vi "old tests.vi"() -> ()   [LabVIEW 2018]
uses:
  CCDCamera/CCDCamera.lvclass
  <userlib>/atmcd32d.llb/Shutter_mode typedef.ctl
  <userlib>/atmcd32d.llb/ReadMode_mode typedef.ctl
  <userlib>/atmcd32d.llb/AcquisitionMode_mode typedef.ctl
  TCPIP/TCPIP.lvclass
  <userlib>/atmcd32d.llb/FITS_type typedef.ctl
  Simulated_CCD_Camera/Simulated_CCD_Camera.lvclass
  Interface/Interface.lvclass
  <userlib>/gfitsio/gfitsio.lvlib
  <userlib>/gfitsio/cfitsio-bitpix.ctl
  C:/Users/observer/Desktop/SPARC4_ACS/SPARC4_ACS/Simulated_CCD_Camera/Simulated_CCD_Camera.lvclass
  <vilib>/Enthought/Python Integration Toolkit/Python Integration Toolkit.lvlib
  <vilib>/Enthought/Python Integration Toolkit/api/Unpack String.vi
  <userlib>/gfitsio/gfitsio-write-image-subset-variant.vi
panel:
  out "error out 7":errorcluster
  in  "Previous CCD Config 2":T4={"PREAMP"=enum."Gain 1", "READOUT_RATE"=enum."1 MHz", "EM_GAIN"=2, "VBIN"=1, "INITIAL_LINE"=1, "INITIAL_COLUMN"=1, "FINAL_LINE"=1024, "FINAL_COLUMN"=1024, "TRIGGER_MODE"=enum."Internal", "HBIN"=1, "SHUTTER_TTL"=enum."TTL Low", "SHUTTER_MODE"=enum."Close", "SHUTTER_OPENING_TIME"=50, "SHUTTER_CLOSING_TIME"=50, "VERTICAL_SHIFT_SPEED"=3, "READ_MODE"=enum."Image", "FRAME_TRANSFER"=TRUE, "VERTICAL_CLOCK_VOLTAGE"=enum."0", "ACQUISITION_MODE"=enum."Kinetics", "AD_CHANNEL"=0, "EM_MODE"=enum."Electron Multiplying"}
  in  "Previous SET parameters 2":T5={"COOLER_POWER_STATUS"=0, "TEMP"=20, "EXPTIME"=1.0, "#FRAMES"=1, "#CUBES"=1}
  out "error out 6":errorcluster
  out "Array":string[](array[string])
  out "Value":string
  out "error out 5":errorcluster
  out "data out":string
  out "Message":string
  out "error out 4":errorcluster
  out "error out 3":errorcluster
  in  "TCPIP in":refnum<class "TCPIP.lvclass">
  out "error out 2":errorcluster
  out "error out":errorcluster
  in  "Previous SET parameters":T5
  in  "Previous CCD Config":T4={"PREAMP"=enum."Gain 1", "READOUT_RATE"=enum."1 MHz", "EM_GAIN"=2, "VBIN"=1, "INITIAL_LINE"=1, "INITIAL_COLUMN"=1, "FINAL_LINE"=1024, "FINAL_COLUMN"=1024, "TRIGGER_MODE"=enum."Internal", "HBIN"=1, "SHUTTER_TTL"=enum."TTL Low", "SHUTTER_MODE"=enum."Close", "SHUTTER_OPENING_TIME"=50, "SHUTTER_CLOSING_TIME"=50, "VERTICAL_SHIFT_SPEED"=3, "READ_MODE"=enum."Image", "FRAME_TRANSFER"=TRUE, "VERTICAL_CLOCK_VOLTAGE"=enum."0", "ACQUISITION_MODE"=enum."Kinetics", "AD_CHANNEL"=0, "EM_MODE"=enum."Electron Multiplying"}
  in  "CCDCamera.lvclass":refnum<class "CCDCamera.lvclass">
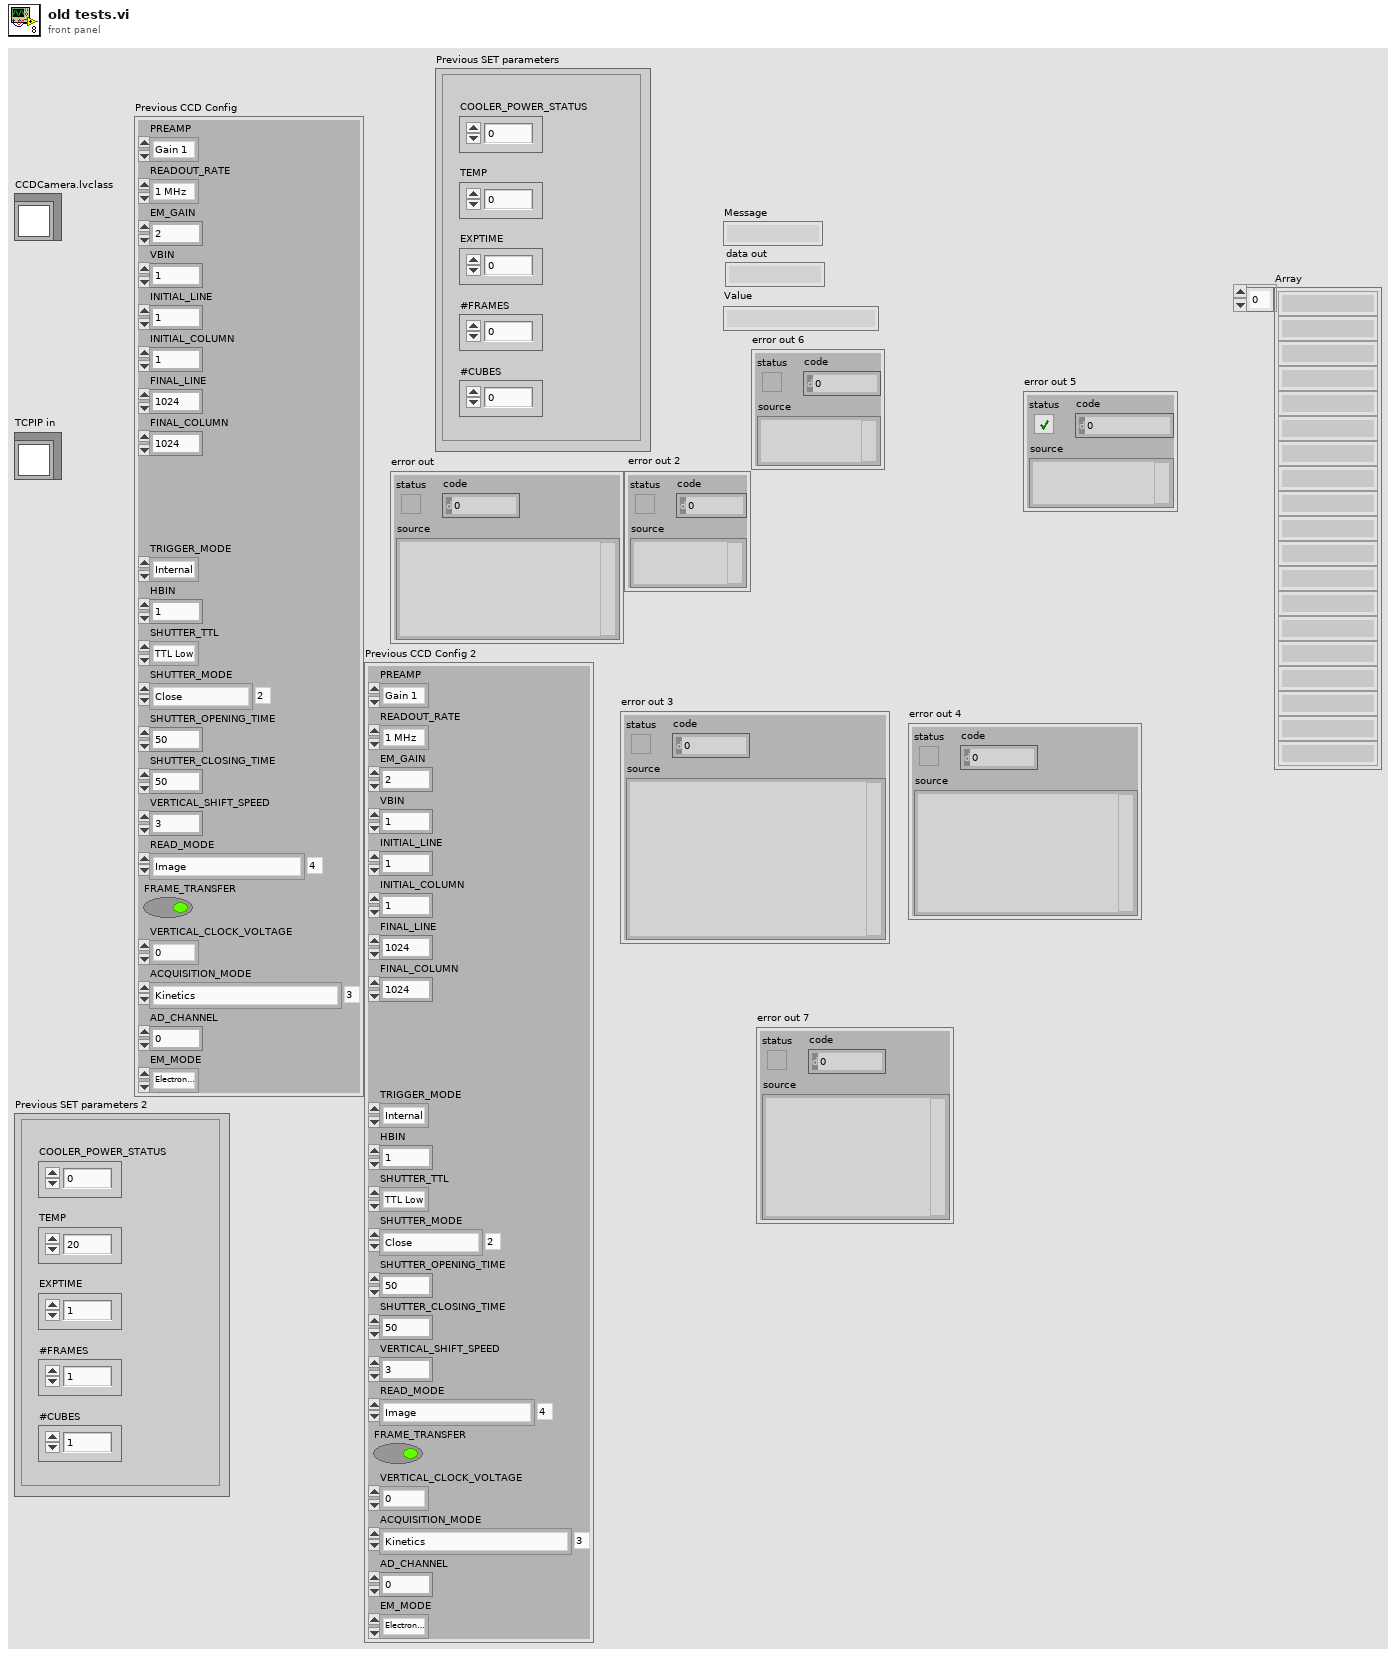
[diagram p1: front panel]
types:
  T1 = typedef "Shutter_mode typedef.ctl" = enum16{"Auto", "Open", "Close", "N/A (3)", "Open FVB Series", "Open Any Series"}
  T2 = typedef "ReadMode_mode typedef.ctl" = enum16{"Full Vertical Binning", "Multi-Track", "Random-Track", "Single-Track", "Image"}
  T3 = typedef "AcquisitionMode_mode typedef.ctl" = enum16{"Reserved (0)", "Single Scan", "Accumulate", "Kinetics", "Fast Kinetics", "Run Till Abort", "Reserved (6)", "Reserved (7)", "Reserved (8)", "Time Delayed Integration"}
  T4 = cluster{"PREAMP":enum16{"Gain 1", "Gain 2"}, "READOUT_RATE":enum16{"30 MHz", "20 MHz", "10 MHz", "1 MHz"}, "EM_GAIN":u16, "VBIN":u16, "INITIAL_LINE":u16, "INITIAL_COLUMN":u16, "FINAL_LINE":u16, "FINAL_COLUMN":u16, "TRIGGER_MODE":enum16{"Internal", "External", "N/A", "N/A_1", "N/A_2", "N/A_3", "External Start"}, "HBIN":u16, "SHUTTER_TTL":enum16{"TTL Low", "TTL High"}, "SHUTTER_MODE":T1, "SHUTTER_OPENING_TIME":u16, "SHUTTER_CLOSING_TIME":u16, "VERTICAL_SHIFT_SPEED":u16, "READ_MODE":T2, "FRAME_TRANSFER":bool, "VERTICAL_CLOCK_VOLTAGE":enum16{"0", "+1", "+2", "+3", "+4"}, "ACQUISITION_MODE":T3, "AD_CHANNEL":u16, "EM_MODE":enum16{"Electron Multiplying", "Conventional"}}
  T5 = cluster{"COOLER_POWER_STATUS":u16, "TEMP":i32, "EXPTIME":dbl, "#FRAMES":u32, "#CUBES":u32}
  T6 = typedef "FITS_type typedef.ctl" = enum16{"Unsigned 16", "Unsigned 32", "Signed 16", "Signed 32", "Float"}
  T7 = enum16{"open", "open or create", "create or replace", "create", "open (read only)"}
  T8 = typedef "gfitsio.lvlib/cfitsio-bitpix.ctl" = i32
  T9 = typedef "gfitsio.lvlib/gfitsio-refnum.ctl" = refnum<k1>
  T10 = enum16{"Standard", "Buffered", "CRLF", "Immediate"}
  T11 = typedef "Python Integration Toolkit.lvlib/Session ID.ctl" = u64
  T12 = typedef "Python Integration Toolkit.lvlib/Python Objects.ctl" = variant
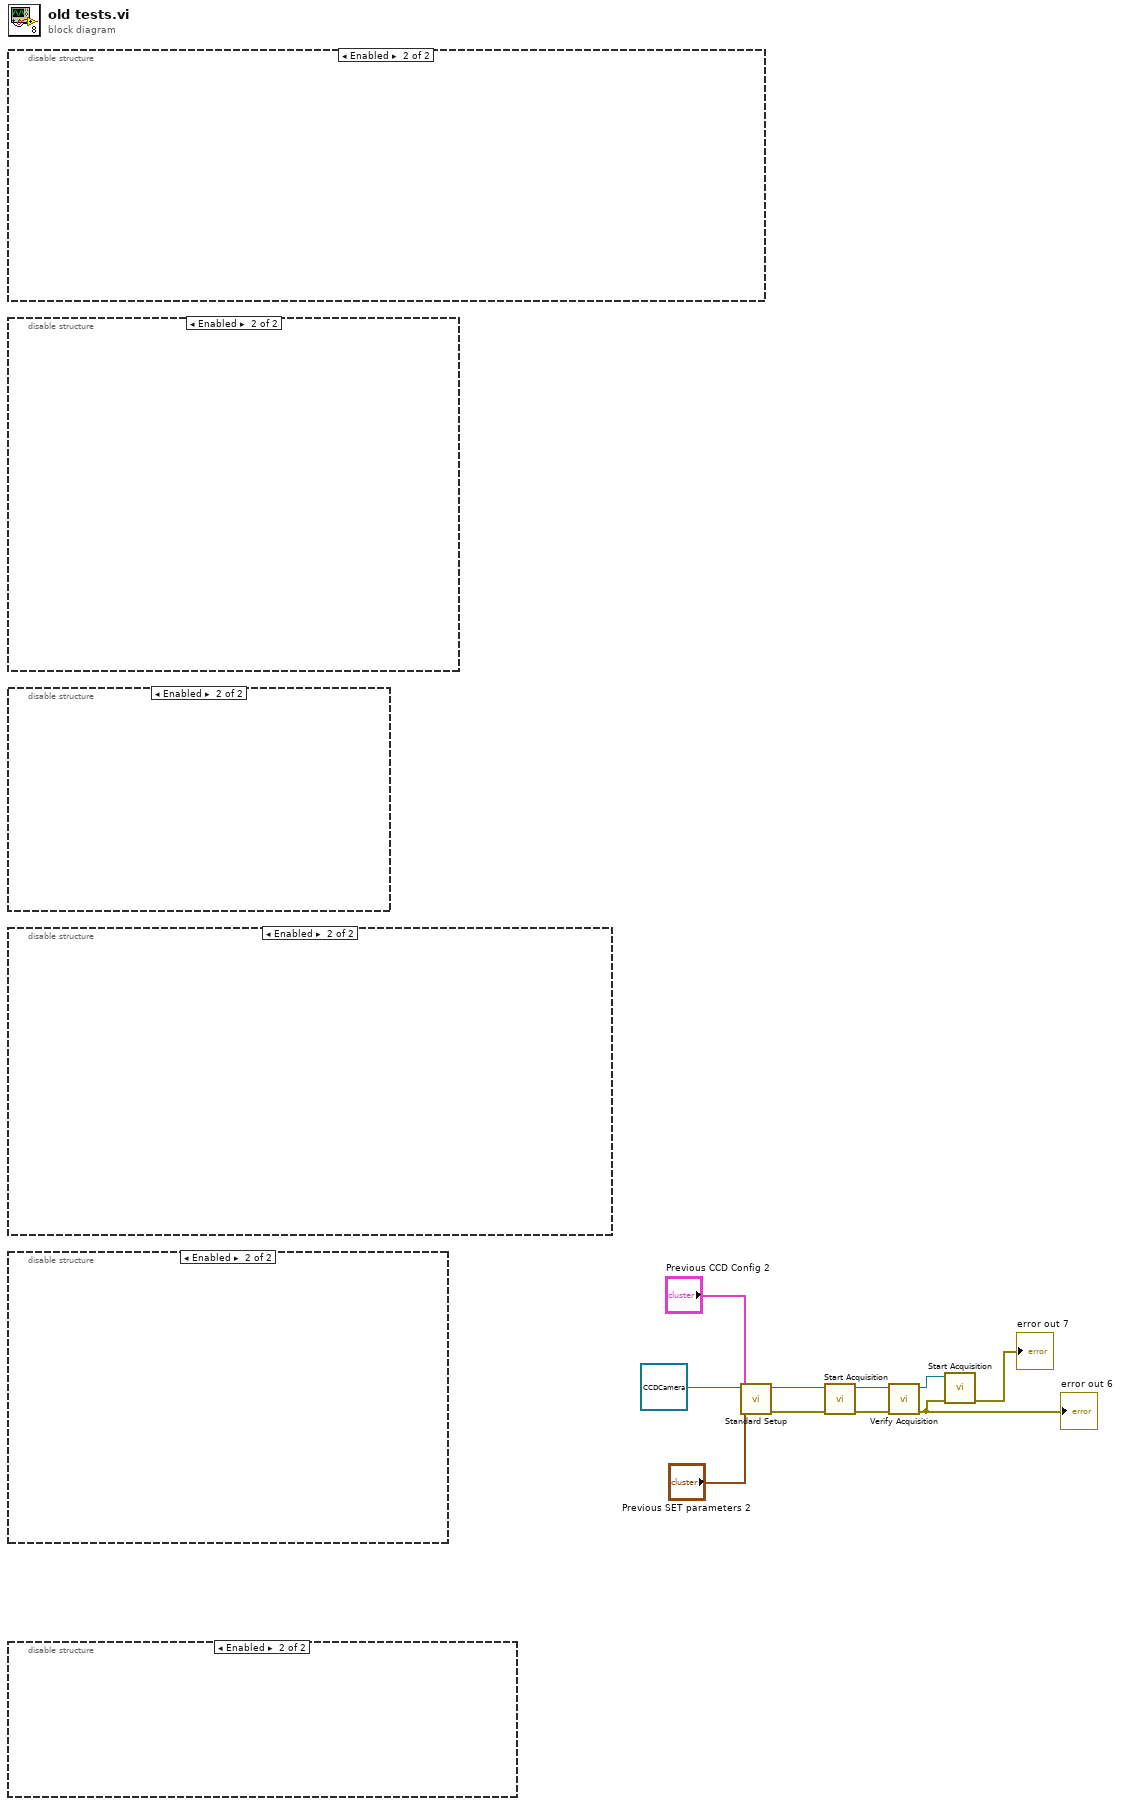
[diagram p0: block diagram]
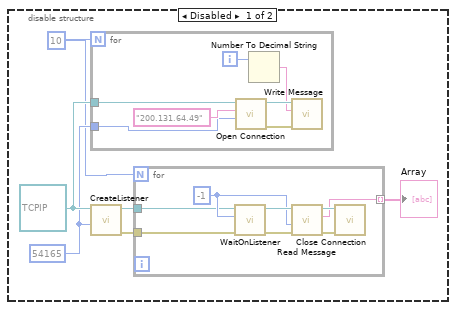
[diagram p2: hidden frame]
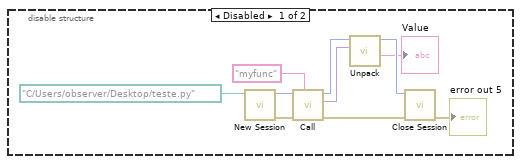
[diagram p3: hidden frame]
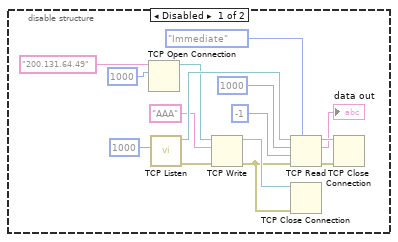
[diagram p4: hidden frame]
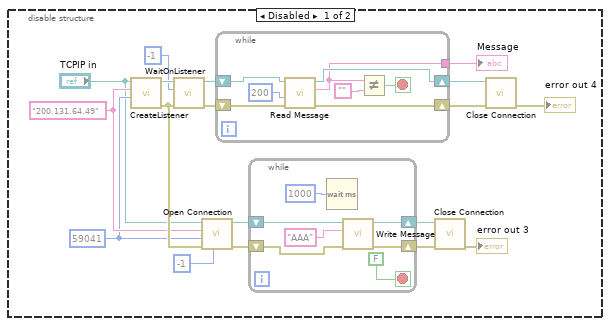
[diagram p5: hidden frame]
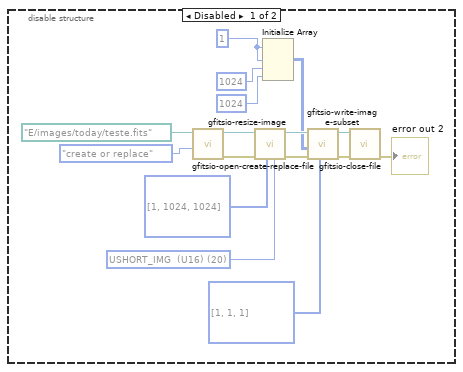
[diagram p6: hidden frame]
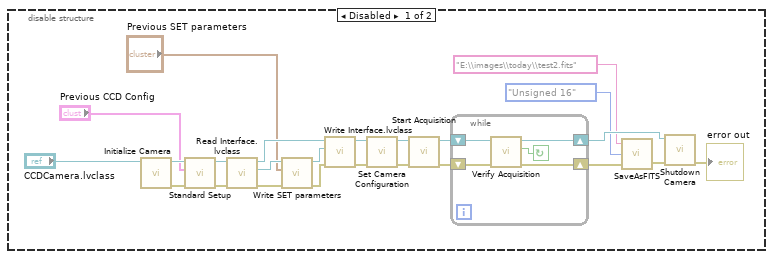
[diagram p7: hidden frame]
diagram:
  n1 = disable-structure shown="Enabled" {
    frame Disabled {
      n2 = call-dynamic "Initialize Camera.vi"("CCDCamera in"="CCDCamera.lvclass") -> ("error out"=w30:errorcluster, "CCDCamera out"=w34:refnum<class "CCDCamera.lvclass">)  [unwired: 9 in]
      n3 = call-dynamic "Standard Setup.vi"("error in (no error)"=w30, "Previous CCD Config"="Previous CCD Config", "CCDCamera in"=w34) -> ("error out"=w21:errorcluster, "CCDCamera out"=w25:refnum<class "CCDCamera.lvclass">)  [unwired: 7 in]
      n4 = call "Read Interface.lvclass.vi"("error in (no error)"=w21, "Simulated_CCD_Camera in"=w25) -> ("error out"=w20:errorcluster, "Interface.lvclass"=w17:refnum<class "Interface.lvclass">, "Simulated_CCD_Camera out"=w24:refnum<class "CCDCamera.lvclass">)  [unwired: 7 in]
      n5 = call "Write SET parameters.vi"("error in (no error)"=w20, "SET parameters"="Previous SET parameters", "Interface in"=w17) -> ("error out"=w19:errorcluster, "Interface out"=w18:refnum<class "Interface.lvclass">)  [unwired: 7 in]
      n6 = call "Write Interface.lvclass.vi"("error in (no error)"=w19, "Interface.lvclass"=w18, "Simulated_CCD_Camera in"=w24) -> ("error out"=w22:errorcluster, "Simulated_CCD_Camera out"=w23:refnum<class "CCDCamera.lvclass">)  [unwired: 7 in]
      n7 = call-dynamic "Set Camera Configuration.vi"("error in (no error)"=w22, "CCDCamera in"=w23) -> ("error out"=w26:errorcluster, "CCDCamera out"=w27:refnum<class "CCDCamera.lvclass">)  [unwired: 8 in]
      n8 = call-dynamic "Start Acquisition.vi"("error in (no error)"=w26, "CCDCamera in"=w27) -> ("error out"=w31:errorcluster, "CCDCamera out"=w33:refnum<class "CCDCamera.lvclass">)  [unwired: 8 in]
      n9 = while {
        shift-right: [w38] -> w32
        shift-left: w33 -> [w39]
        shift-right: [w35] -> w11
        shift-left: w31 -> [w37]
        stop <- w36 continue-if-true
        n10 = call-dynamic "Verify Acquisition.vi"("error in (no error)"=w37, "CCDCamera in"=w39) -> ("error out"=w35:errorcluster, "Acquiring"=w36:bool, "CCDCamera out"=w38:refnum<class "CCDCamera.lvclass">)  [unwired: 7 in]
      }
      n11 = call <userlib>:"SaveAsFITS.vi"("error in (no error)"=w11, "FITS_type"=FITS_type_typedef."Unsigned 16", "path"="E:\\images\\today\\test2.fits") -> ("error out"=w12:errorcluster)  [unwired: 1 out]
      n12 = call-dynamic "Shutdown Camera.vi"("error in (no error)"=w12, "CCDCamera in"=w32) -> ("error out"=→"error out":errorcluster)  [unwired: 8 in, 1 out]
    }
    frame Enabled {
    }
  }
  n13 = disable-structure shown="Enabled" {
    frame Disabled {
      w45 = 1 ("dimension size")
      w48 = T8 20 items=["<invalid type>"=0, "BYTE_IMG  (U8)"=8, "SHORT_IMG  (I16)"=16, "USHORT_IMG  (U16)"=20, "LONG_IMG  (I32)"=32, "ULONG_IMG  (U32)"=40, "FLOAT_IMG  (SGL)"=-32, "DOUBLE_IMG  (DBL)"=-64] ("image data type")
      n14 = call <userlib>:"gfitsio-open-create-replace-file.vi"("function (open)"=T7."create or replace", "file path (dialog if empty)"=path "E:/images/today/teste.fits") -> ("error out"=w50:errorcluster, "gfits refnum"=w55:T9)  [unwired: 7 in, 1 out]
      n15 = call <userlib>:"gfitsio-resize-image.vi"("image data type"=w48, "naxes"=i32[] [1, 1024, 1024], "error in (no error)"=w50, "gfits refnum"=w55) -> ("error out"=w51:errorcluster, "dup gfits refnum"=w54:T9)  [unwired: 6 in]
      n16 = Initialize Array(w45, w45, 1024 ("dimension size"), 1024 ("dimension size")) -> (w44:i32[][][])
      n17 = call-poly <userlib>:"gfitsio-write-image-subset.vi"("fpixel"=i32[] [1, 1, 1] ("naxes"), "error in (no error)"=w51, "data"=w44, "gfits refnum"=w54) -> ("error out"=w52:errorcluster, "dup gfits refnum"=w53:T9)  [unwired: 6 in]
      n18 = call <userlib>:"gfitsio-close-file.vi"("error in (no error)"=w52, "gfits refnum"=w53) -> ("error out"=→"error out 2":errorcluster)  [unwired: 8 in, 1 out]
    }
    frame Enabled {
    }
  }
  n19 = disable-structure shown="Enabled" {
    frame Disabled {
      n20 = TCP Open Connection(address="200.131.64.49", remote port or service name=u16 1000) -> (connection ID=w64:refnum<k5>)  [unwired: 3 in, 1 out]
      n21 = call <vilib>:"TCP Listen.vi"("port"=u16 1000) -> ("error out"=w59:errorcluster, "connection ID"=w69:refnum<k5>)  [unwired: 6 in, 3 out]
      n22 = TCP Write(connection ID=w64, data in="AAA", error in (no error)=w59) -> (connection ID out=w63:refnum<k5>, error out=w58:errorcluster)  [unwired: 1 in, 1 out]
      n23 = TCP Read(connection ID=w69, bytes to read=1000, error in (no error)=w58, 7:T10."Immediate" ("mode (standard)"), 9:-1 ("timeout ms (25000)")) -> (connection ID out=w68:refnum<k5>, data out=→"data out":string, error out=w67:errorcluster)
      n24 = TCP Close Connection(connection ID=w63, error in (no error)=w58) -> ()  [unwired: 1 in, 2 out]
      n25 = TCP Close Connection(connection ID=w68, error in (no error)=w67) -> ()  [unwired: 1 in, 2 out]
    }
    frame Enabled {
    }
  }
  n26 = disable-structure shown="Enabled" {
    frame Disabled {
      w85 = u16 59041 ("remote port")
      w86 = "200.131.64.49" ("IP")
      n27 = call-dynamic "CreateListener.vi"("remote port"=w85, 10:w86, "TCPIP in"="TCPIP in") -> ("error out"=w87:errorcluster, "TCPIP out"=w88:refnum<class "TCPIP.lvclass">)  [unwired: 7 in]
      n28 = call-dynamic "WaitOnListener.vi"("error in (no error)"=w87, "timeout ms"=-1, "TCPIP in"=w88) -> ("error out"=w76:errorcluster, "TCPIP out"=w77:refnum<class "TCPIP.lvclass">)  [unwired: 7 in]
      n29 = call "Open Connection.vi"("timeout"=-1, "error in (no error)"=w87, "remote port"=w85, "IP"=w86, "TCPIP in"="TCPIP in") -> ("error out"=w78:errorcluster, "TCPIP out"=w81:refnum<class "TCPIP.lvclass">)  [unwired: 5 in]
      n30 = while {
        tunnel: [w90] -> w72
        shift-right: [w92] -> w74
        shift-left: w77 -> [w96]
        shift-right: [w93] -> w75
        shift-left: w76 -> [w95]
        stop <- w91 stop-if-true
        n31 = call "Read Message.vi"("error in (no error)"=w95, "timeout"=200, "TCPIP in"=w96) -> ("error out"=w93:errorcluster, "Message"=w90:string, "TCPIP out"=w92:refnum<class "TCPIP.lvclass">)  [unwired: 6 in]
        n32 = Not Equal?(x=w90, y="") -> (x != y?=w91:bool)
      }
      "Message" <- w72
      n33 = while {
        shift-right: [w102] -> w80
        shift-left: w81 -> [w103]
        shift-right: [w101] -> w79
        shift-left: w78 -> [w100]
        stop <- FALSE stop-if-true
        n34 = Wait (ms)(milliseconds to wait=u32 1000) -> ()  [unwired: 1 out]
        n35 = call "Write Message.vi"("error in (no error)"=w100, "Message"="AAA", "TCPIP in"=w103) -> ("error out"=w101:errorcluster, "TCPIP out"=w102:refnum<class "TCPIP.lvclass">)  [unwired: 7 in]
      }
      n36 = call "Close Connection.vi"("error in (no error)"=w79, "TCPIP in"=w80) -> ("error out"=→"error out 3":errorcluster)  [unwired: 8 in, 1 out]
      n37 = call "Close Connection.vi"("error in (no error)"=w75, "TCPIP in"=w74) -> ("error out"=→"error out 4":errorcluster)  [unwired: 8 in, 1 out]
    }
    frame Enabled {
    }
  }
  n38 = disable-structure shown="Enabled" {
    frame Disabled {
      w104 = 10
      w108 = u16 54165 ("remote port")
      w109 = refnum<class "TCPIP.lvclass"> refnum ("TCPIP.lvclass")
      n39 = for {
        N: w104 -> [_]
        tunnel: w109 -> [w121]
        tunnel: w108 -> [w120]
        i -> [w119]
        n40 = call "Open Connection.vi"("remote port"=w120, "IP"="200.131.64.49", "TCPIP in"=w121) -> ("error out"=w122:errorcluster, "TCPIP out"=w123:refnum<class "TCPIP.lvclass">)  [unwired: 7 in]
        n41 = Number To Decimal String(number=w119) -> (decimal integer string=w118:string)  [unwired: 1 in]
        n42 = call "Write Message.vi"("error in (no error)"=w122, "Message"=w118, "TCPIP in"=w123) -> ()  [unwired: 7 in, 2 out]
      }
      n43 = call-dynamic "CreateListener.vi"("remote port"=w108, "TCPIP in"=w109) -> ("error out"=w107:errorcluster, "TCPIP out"=w106:refnum<class "TCPIP.lvclass">)  [unwired: 8 in]
      n44 = for {
        N: w104 -> [_]
        tunnel: w107 -> [w112]
        tunnel: w106 -> [w111]
        tunnel: [w110] -> w105 mode=indexing
        w115 = -1 ("timeout ms")
        n45 = call-dynamic "WaitOnListener.vi"("error in (no error)"=w112, "timeout ms"=w115, "TCPIP in"=w111) -> ("error out"=w116:errorcluster, "TCPIP out"=w117:refnum<class "TCPIP.lvclass">)  [unwired: 7 in]
        n46 = call "Read Message.vi"("error in (no error)"=w116, "timeout"=w115, "TCPIP in"=w117) -> ("error out"=w113:errorcluster, "Message"=w110:string, "TCPIP out"=w114:refnum<class "TCPIP.lvclass">)  [unwired: 6 in]
        n47 = call "Close Connection.vi"("error in (no error)"=w113, "TCPIP in"=w114) -> ()  [unwired: 8 in, 2 out]
      }
      "Array" <- w105
    }
    frame Enabled {
    }
  }
  n48 = disable-structure shown="Enabled" {
    frame Disabled {
      n49 = call <vilib>:"New Session.vi"("Path to Python Module (.py File)"=path "C:/Users/observer/Desktop/teste.py") -> ("error out"=w131:errorcluster, "Session ID out"=w132:T11)  [unwired: 9 in]
      n50 = call <vilib>:"Call.vi"("Function or Method Name"="myfunc", "error in (no error)"=w131, "Session ID"=w132) -> ("error out"=w130:errorcluster, "Python Object References Out"=w127:T12, "Session ID out"=w128:T11)  [unwired: 6 in]
      n51 = call-poly <vilib>:"Unpack.vi"("Python Object References In"=w127, "Session ID"=w128) -> ("Value"=→"Value":string, "Session ID out"=w126:T11)  [unwired: 6 in, 2 out]
      n52 = call <vilib>:"Close Session.vi"("error in (no error)"=w130, "Session ID"=w126) -> ("error out"=→"error out 5":errorcluster)  [unwired: 9 in]
    }
    frame Enabled {
    }
  }
  n53 = call-dynamic "Standard Setup.vi"("Previous SET parameters"="Previous SET parameters 2", "Previous CCD Config"="Previous CCD Config 2", "CCDCamera in"=refnum<class "CCDCamera.lvclass"> refnum ("CCDCamera.lvclass")) -> ("error out"=w4:errorcluster, "CCDCamera out"=w5:refnum<class "CCDCamera.lvclass">)  [unwired: 7 in]
  n54 = call-dynamic "Start Acquisition.vi"("error in (no error)"=w4, "CCDCamera in"=w5) -> ("error out"=w6:errorcluster, "CCDCamera out"=w10:refnum<class "CCDCamera.lvclass">)  [unwired: 8 in]
  n55 = call-dynamic "Verify Acquisition.vi"("error in (no error)"=w6, "CCDCamera in"=w10) -> ("error out"=w3:errorcluster, "CCDCamera out"=w2:refnum<class "CCDCamera.lvclass">)  [unwired: 7 in, 1 out]
  "error out 6" <- w3
  n56 = call-dynamic "Start Acquisition.vi"("error in (no error)"=w3, "CCDCamera in"=w2) -> ("error out"=→"error out 7":errorcluster)  [unwired: 8 in, 1 out]
